vi "Extract the Sine Wave.vi"() -> ()   [LabVIEW 2020]
doc: "This example demonstrates how a signal can be extracted from bandlimited noise using the filter VIs."
uses:
  <vilib>/Analysis/3filter.llb/Filter Passband Type.ctl
  <vilib>/Analysis/3filter.llb/Butterworth Filter (DBL).vi
  <vilib>/Analysis/NI_AALBase.lvlib
panel:
  in  "Sample rate (Hz)":dbl=1000.0
  out "Signals":cluster{dbl, dbl, "Filtered X":dbl[]}[](graph)
  in  "Stop":bool
  in  "Filter Order":i32(slide)=5 scale=0.0..10.0
  in  "Cut-Off Frequency (Hz)":dbl(slide)=20.0 scale=0.0..100.0
  in  "Sine Frequency (Hz)":dbl(slide)=10.0 scale=0.0..10.0
  # "Overview: Removes additive noise from a sinusoid using a lowpass filter.\nRequirements: LabVIEW Full Development System\nInstructions:\n1. Run the VI.\n2. Change the Cut-Off Frequency and Filter Order, noting the effect on the filtered waveform.\n3. Click Stop to stop the VI."
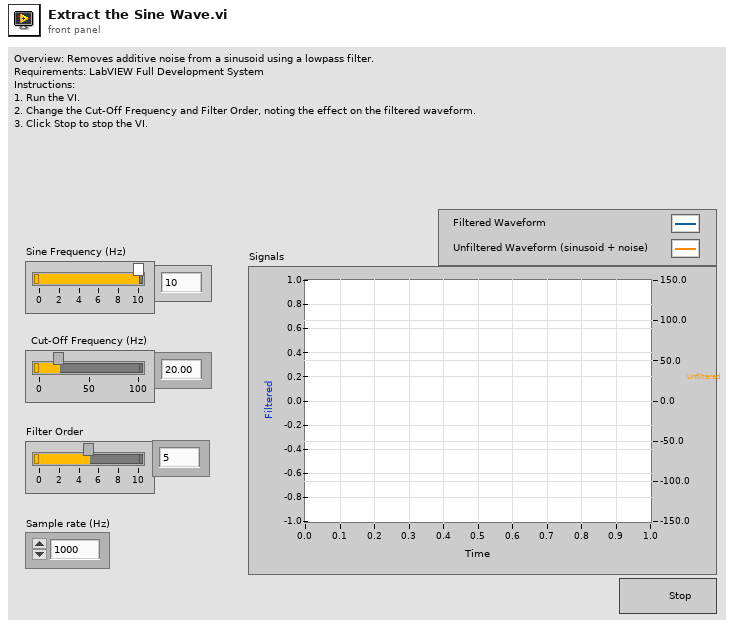
[diagram p1: front panel]
types:
  T1 = typedef "NI_AALBase.lvlib/Filter Passband Type.ctl" = enum32{"Lowpass", "Highpass", "Bandpass", "Bandstop"}
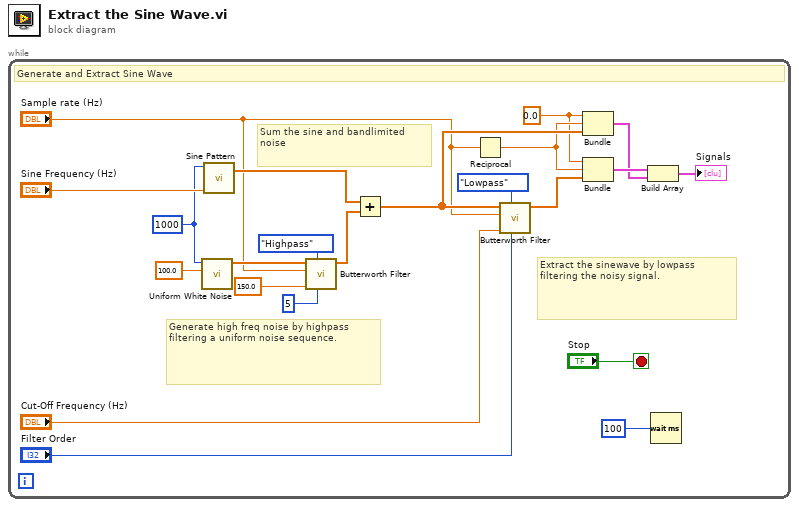
[diagram p0: block diagram]
diagram:
  n1 = while {
    stop <- "Stop" stop-if-true
    w4 = 1000
    w6 = 0.0
    # "Extract the sinewave by lowpass filtering the noisy signal."
    # "Sum the sine and bandlimited noise"
    # "Generate high freq noise by highpass filtering a uniform noise sequence."
    # "Generate and Extract Sine Wave"
    n2 = call <vilib>:"Uniform White Noise.vi"("amplitude"=100.0, "samples"=w4) -> ("uniform white noise"=w21:dbl[])  [unwired: 8 in, 1 out]
    n3 = call <vilib>:"Sine Pattern.vi"("cycles"="Sine Frequency (Hz)", "samples"=w4) -> ("Sinusoidal Pattern"=w19:dbl[])  [unwired: 2 in, 1 out]
    n4 = call-poly <vilib>:"Butterworth Filter.vi"("order"=5, "filter type"=Filter_Passband_Type."Highpass", "low cutoff freq: fl"=150.0, "sampling freq: fs"="Sample rate (Hz)", "X"=w21) -> ("Filtered X"=w20:dbl[])  [unwired: 3 in, 1 out]
    n5 = Add(x=w19, y=w20) -> (x+y=w15:dbl[])
    n6 = Reciprocal(x="Sample rate (Hz)") -> (1/x=w14:dbl)
    n7 = call-poly <vilib>:"Butterworth Filter.vi"("order"="Filter Order", "filter type"=Filter_Passband_Type."Lowpass", "low cutoff freq: fl"="Cut-Off Frequency (Hz)", "sampling freq: fs"="Sample rate (Hz)", "X"=w15) -> ("Filtered X"=w16:dbl[])  [unwired: 3 in, 1 out]
    n8 = Bundle(w6, w14, w15) -> (w11:cluster{dbl, dbl, dbl[]})  [unwired: 1 in]
    n9 = Bundle(w6, w14, "Filtered X"=w16) -> (w12:cluster{dbl, dbl, "Filtered X":dbl[]})  [unwired: 1 in]
    n10 = Build Array(w12, w11) -> (→"Signals":cluster{dbl, dbl, "Filtered X":dbl[]}[])
    n11 = Wait (ms)(milliseconds to wait=u32 100) -> ()  [unwired: 1 out]
  }
